vi "5.feladat.vi"() -> ()   [LabVIEW 2015]
panel:
  out "difference between LED and button press in ms":dbl
  in  "?":bool
  out "current ms":dbl
  out "random ms":dbl
  out "?":bool
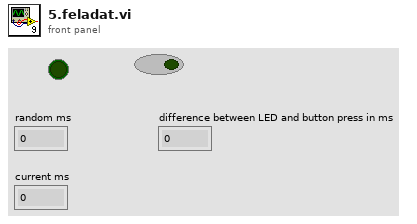
[diagram p1: front panel]
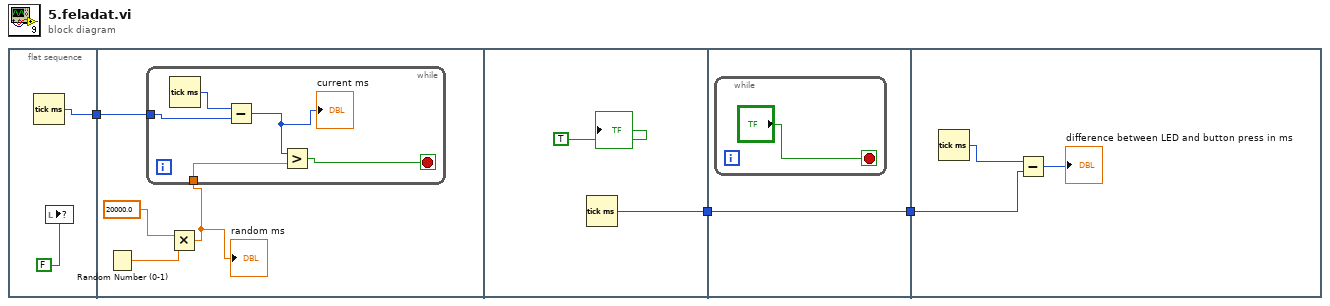
[diagram p0: block diagram]
diagram:
  n1 = flat-sequence {
    tunnel: [w5] -> w3
    tunnel: w3 -> [w7]
    tunnel: [w15] -> w1
    tunnel: [w17] -> w2
    tunnel: w1 -> [w17]
    tunnel: w2 -> [w20]
    frame #0 {
      n2 = Tick Count (ms)() -> (millisecond timer value=w5:u32)
      n3 = local write item#?(FALSE) -> ()
    }
    frame #1 {
      n4 = Random Number (0-1)() -> (number: 0 to 1=w8:dbl)
      n5 = Multiply(x=20000.0, y=w8) -> (x*y=w6:dbl)
      "random ms" <- w6
      n6 = while {
        tunnel: w7 -> [w13]
        tunnel: w6 -> [w12]
        stop <- w11 stop-if-true
        n7 = Tick Count (ms)() -> (millisecond timer value=w14:u32)
        n8 = Subtract(x=w14, y=w13) -> (x-y=w10:u32)
        "current ms" <- w10
        n9 = Greater?(x=w10, y=w12) -> (0:w11:bool)
      }
    }
    frame #2 {
      n10 = Tick Count (ms)() -> (millisecond timer value=w15:u32)
      "?" <- TRUE
    }
    frame #3 {
      n11 = while {
        stop <- "?" stop-if-true
      }
    }
    frame #4 {
      n12 = Tick Count (ms)() -> (millisecond timer value=w21:u32)
      n13 = Subtract(x=w21, y=w20) -> (x-y=→"difference between LED and button press in ms":u32)
    }
  }
